vi "CAENHV Set Sys Prop String.vi"(8 "error in (no error)":errorcluster, 9 "Set":string, 10 "PropName":string, 11 "handle":i32) -> (0 "error out":errorcluster)   [LabVIEW 2018, in "CAENHVWrapper.lvlib"]
doc: "CAENHVLIB_API CAENHVRESULT CAENHV_SetSysProp(int handle, \n const char *PropName, void *Set);"
uses:
  <instrlib>/CAENHVWrapper/CAENHVWrapper.lvlib
  <instrlib>/CAENHVWrapper/VIs/CAENHVWrapper.dll
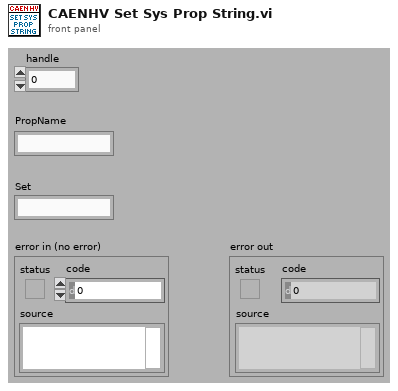
[diagram p1: front panel]
types:
  T1 = typedef "CAENHVWrapper.lvlib/SYSPROP_TYPE.ctl" = enum32{"SYSPROP_TYPE_STR", "SYSPROP_TYPE_REAL", "SYSPROP_TYPE_UINT2", "SYSPROP_TYPE_UINT4", "SYSPROP_TYPE_INT2", "SYSPROP_TYPE_INT4", "SYSPROP_TYPE_BOOLEAN"}
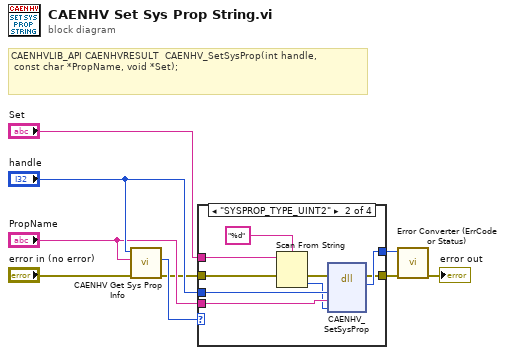
[diagram p0: block diagram]
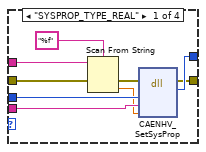
[diagram p2: hidden frame]
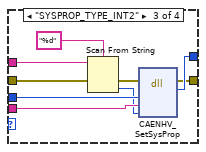
[diagram p3: hidden frame]
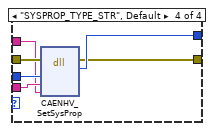
[diagram p4: hidden frame]
diagram:
  # "CAENHVLIB_API CAENHVRESULT  CAENHV_SetSysProp(int handle, \n const char\t*PropName, void *Set);"
  n1 = call <instrlib>:"CAENHV Get Sys Prop Info.vi"("error in (no error)"="error in (no error)", "PropName"="PropName", "handle"="handle") -> ("error out"=w2:errorcluster, "PropType"=w3:T1)  [unwired: 6 in, 1 out]
  n2 = case shown="\"SYSPROP_TYPE_UINT2\"" w3 {
    tunnel: [w18 w27 w36 w42] -> w9
    tunnel: [w17 w26 w35 w41] -> w8
    tunnel: "handle" -> [w16 w25 w34 w40]
    tunnel: "PropName" -> [w15 w24 w33 w39]
    tunnel: w2 -> [w14 w23 w32 w38]
    tunnel: "Set" -> [w10 w19 w28 w37]
    frame "SYSPROP_TYPE_REAL" {
      n3 = Scan From String(format string="%f", input string=w10, error in=w14) -> (error out=w13:errorcluster, output 1=w12:dbl)  [unwired: 2 in, 2 out]
      n4 = dll-call lib="C:/Program Files (x86)/National Instruments/LabVIEW 2018/instr.lib/CAENHVWrapper/VIs/CAENHVWrapper.*" fn="CAENHV_SetSysProp"(error in=w13, "handle"=w16, "PropName"=w15, "Set"=w12) -> (error out=w17:errorcluster, "return type"=w18:i32)  [unwired: 5 in, 1 out]
    }
    frame "SYSPROP_TYPE_UINT2" {
      n5 = Scan From String(format string="%d", input string=w19, error in=w23) -> (error out=w22:errorcluster, output 1=w21:i32)  [unwired: 2 in, 2 out]
      n6 = dll-call lib="C:/Program Files (x86)/National Instruments/LabVIEW 2018/instr.lib/CAENHVWrapper/VIs/CAENHVWrapper.*" fn="CAENHV_SetSysProp"(error in=w22, "handle"=w25, "PropName"=w24, "Set"=w21) -> (error out=w26:errorcluster, "return type"=w27:i32)  [unwired: 5 in, 1 out]
    }
    frame "SYSPROP_TYPE_INT2" {
      n7 = Scan From String(format string="%d", input string=w28, error in=w32) -> (error out=w31:errorcluster, output 1=w30:i32)  [unwired: 2 in, 2 out]
      n8 = dll-call lib="C:/Program Files (x86)/National Instruments/LabVIEW 2018/instr.lib/CAENHVWrapper/VIs/CAENHVWrapper.*" fn="CAENHV_SetSysProp"(error in=w31, "handle"=w34, "PropName"=w33, "Set"=w30) -> (error out=w35:errorcluster, "return type"=w36:u16)  [unwired: 5 in, 1 out]
    }
    frame "SYSPROP_TYPE_STR", Default {
      n9 = dll-call lib="C:/Program Files (x86)/National Instruments/LabVIEW 2018/instr.lib/CAENHVWrapper/VIs/CAENHVWrapper.*" fn="CAENHV_SetSysProp"(error in=w38, "handle"=w40, "PropName"=w39, "Set"=w37) -> (error out=w41:errorcluster, "return type"=w42:u16)  [unwired: 5 in, 1 out]
    }
  }
  n10 = call <instrlib>:"Error Converter (ErrCode or Status).vi"("error in (no error)"=w8, "error code"=w9) -> ("error out"=→"error out":errorcluster)  [unwired: 9 in]
